vi "main.vi"() -> ()   [LabVIEW 2015]
uses:
  BLE Context/BLE context.lvclass
  ctrls/RefsBox.ctl
  ctrls/QData.ctl
  ctrls/States.ctl
  BLE Message/BLE Message.lvclass
  BLE Context/BLE context.lvclass/BLE context.ctl
panel:
  out "In queue:":i32 caption="Numeric"
  out "Accelerometers":cluster{dbl, dbl, dbl}(graph) caption="Body position:"
  out "HRS Plot":u32(graph) caption="Heart Rate: 102"
  out "Device name":string caption="String"
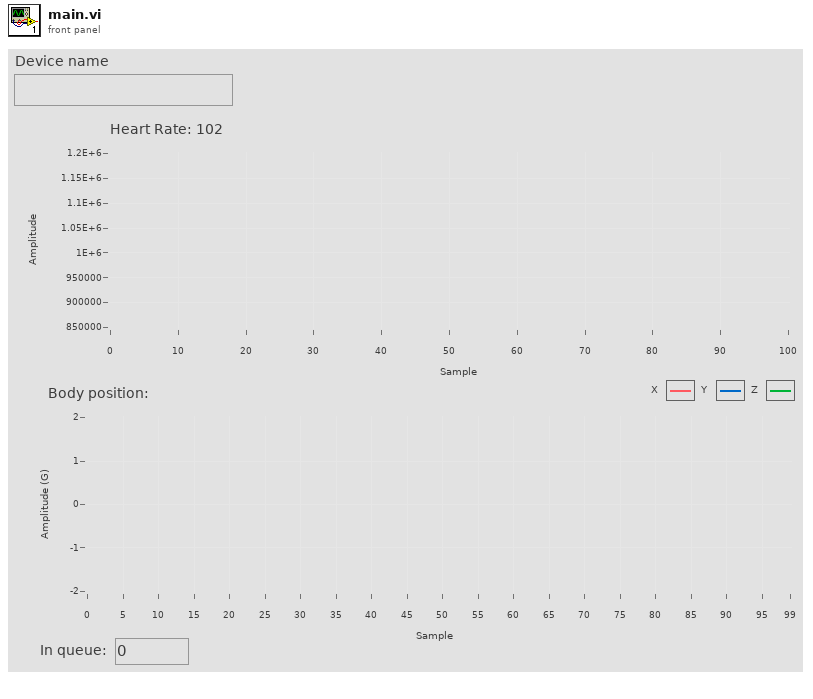
[diagram p1: front panel]
types:
  T1 = typedef "QData.ctl" = cluster{"States":T2, "BLE Message.lvclass":refnum<class "BLE Message.lvclass">}
  T2 = typedef "States.ctl" = enum16{"Stop", "Send"}
  T3 = typedef "RefsBox.ctl" = cluster{"Heart Rate Plot ref":refnum<vi>, "Accelerometers":refnum<vi>, "Main VI":refnum<vi>}
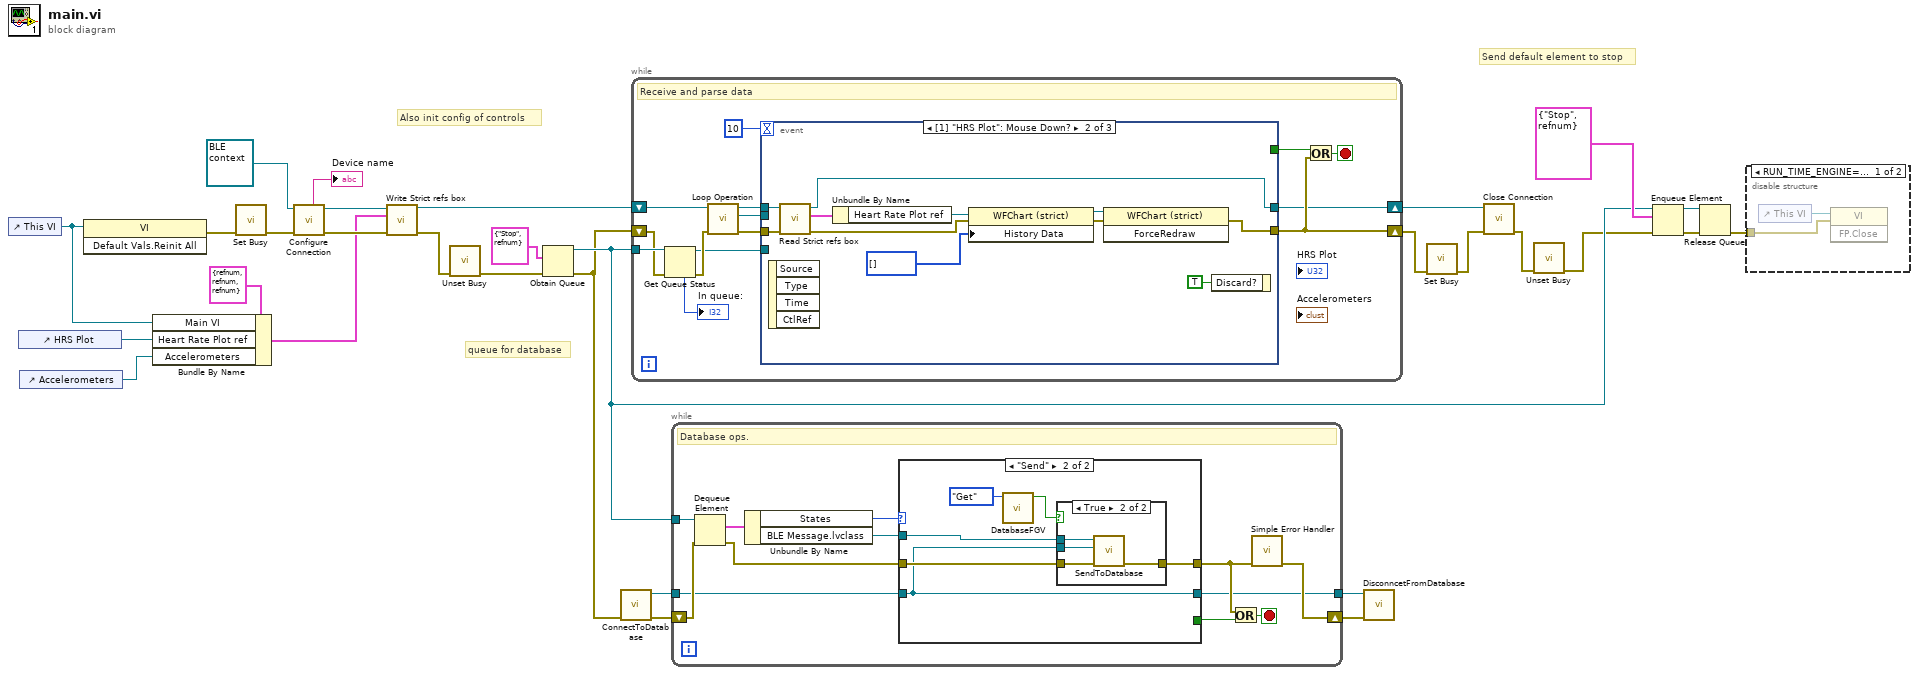
[diagram p0: block diagram]
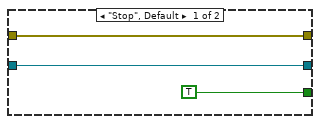
[diagram p3: hidden frame]
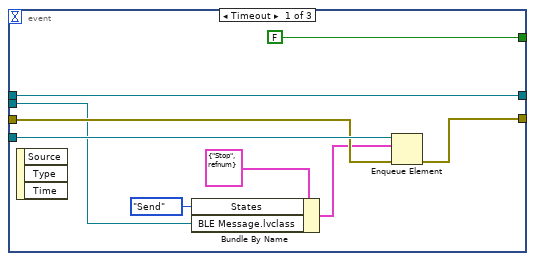
[diagram p5: hidden frame]
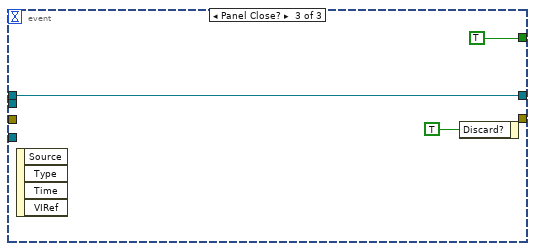
[diagram p6: hidden frame]
diagram:
  # "Send default element to stop"
  # "Also init config of controls"
  # "queue for database"
  n1 = control-ref of="This VI"() -> (w1:refnum<vi>)
  n2 = control-ref of="HRS Plot"() -> (w27:refnum<vi>)
  n3 = control-ref of="Accelerometers"() -> (w21:refnum<vi>)
  n4 = invoke class="VI" method="Default Vals.Reinit All"(reference=w1) -> (error out=w5:errorcluster)  [unwired: 2 in, 2 out]
  n5 = Bundle By Name(cluster=T3 {"Heart Rate Plot ref"=refnum, "Accelerometers"=refnum, "Main VI"=refnum} ("Strict refs box"), "Main VI"=w1, "Heart Rate Plot ref"=w27, "Accelerometers"=w21) -> (w23:T3)
  n6 = call <vilib>:"Set Busy.vi"("error in (no error)"=w5) -> ("error out"=w4:errorcluster)  [unwired: 9 in, 1 out]
  n7 = call "Configure Connection.vi"("error in (no error)"=w4, "BLE context in"=refnum<class "BLE context.lvclass"> refnum ("BLE context.lvclass")) -> ("error out"=w25:errorcluster, "BLE context out"=w26:refnum<class "BLE context.lvclass">, "Device name"=→"Device name":string)  [unwired: 7 in]
  n8 = call "Write Strict refs box.vi"("error in (no error)"=w25, "Strict refs box"=w23, "BLE context in"=w26) -> ("error out"=w3:errorcluster, "BLE context out"=w24:refnum<class "BLE context.lvclass">)  [unwired: 7 in]
  n9 = call <vilib>:"Unset Busy.vi"("error in (no error)"=w3) -> ("error out"=w2:errorcluster)  [unwired: 10 in]
  n10 = Obtain Queue(element data type=T1 {"States"=enum."Stop", "BLE Message.lvclass"=refnum} ("Cluster"), error in (no error)=w2) -> (queue out=w16:refnum<queue>, error out=w14:errorcluster)  [unwired: 3 in, 1 out]
  n11 = call "ConnectToDatabase.vi"("error in"=w14) -> ("error out"=w15:errorcluster, "Database ref"=w13:refnum<k24>)  [unwired: 9 in]
  n12 = while {
    shift-right: [w39] -> w22
    shift-left: w24 -> [w43]
    shift-right: [w40] -> w12
    shift-left: w14 -> [w34]
    tunnel: w16 -> [w35]
    stop <- w44 stop-if-true
    # "Receive and parse data"
    n13 = Get Queue Status(queue=w35, error in (no error)=w34) -> (queue out=w32:refnum<queue>, error out=w33:errorcluster, # elements in queue=→"In queue:":i32)  [unwired: 1 in, 5 out]
    n14 = call "Loop Operation.vi"("error in (no error)"=w33, "BLE context in"=w43) -> ("error out"=w41:errorcluster, "BLE Message out"=w42:refnum<class "BLE Message.lvclass">, "BLE context out"=w38:refnum<class "BLE context.lvclass">)  [unwired: 7 in]
    n15 = event shown="[1] \"HRS Plot\": Mouse Down?" {
      selector: _ -> [_ _ _]
      dyn-events: _ -> [_ _ _]
      timeout: 10 -> [_ _ _]
      tunnel: w42 -> [w47 _ _]
      tunnel: w32 -> [w53 _ _]
      tunnel: w41 -> [w52 w63 _]
      tunnel: [w51 w56 _] -> w40
      tunnel: [w50 w55 w65] -> w39
      tunnel: w38 -> [w50 w64 w65]
      tunnel: [FALSE _ TRUE ("stop? (T)")] -> w36
      event Timeout {
        n16 = event-data() -> ()  [unwired: 1 in, 3 out]
        n17 = Bundle By Name(cluster=T1 {"States"=enum."Stop", "BLE Message.lvclass"=refnum} ("Cluster"), "States"=States."Send", "BLE Message.lvclass"=w47) -> (w45:T1)
        n18 = Enqueue Element(queue=w53, element=w45, error in (no error)=w52) -> (error out=w51:errorcluster)  [unwired: 1 in, 2 out]
      }
      event "HRS Plot": Mouse Down? {
        n19 = event-data() -> ()  [unwired: 1 in, 4 out]
        n20 = call "Read Strict refs box.vi"("error in (no error)"=w63, "BLE context in"=w64) -> ("error out"=w60:errorcluster, "Strict refs box"=w62:T3, "BLE context out"=w55:refnum<class "BLE context.lvclass">)  [unwired: 7 in]
        n21 = Unbundle By Name(w62) -> ("Heart Rate Plot ref"=w61:refnum<vi>)
        n22 = property class="WFChart (strict)"(reference=w61, error in=w60, "History Data"=u32[] []) -> (reference out=w58:refnum<vi>, error out=w57:errorcluster)
        n23 = invoke class="WFChart (strict)" method="ForceRedraw"(reference=w58, error in=w57) -> (error out=w56:errorcluster)  [unwired: 1 in, 2 out]
        n24 = event-data("Discard?"=TRUE) -> ()  [unwired: 1 in, 1 out]
      }
      event Panel Close? {
        n25 = event-data() -> ()  [unwired: 1 in, 4 out]
        n26 = event-data("Discard?"=TRUE) -> ()  [unwired: 1 in, 1 out]
      }
    }
    n27 = Or(x=w36, y=w40) -> (x .or. y?=w44:bool)
  }
  n28 = while {
    tunnel: w16 -> [w79]
    shift-right: [w73] -> w7
    shift-left: w15 -> [w78]
    tunnel: w13 -> [w69]
    tunnel: [w68] -> w8
    stop <- w72 stop-if-true
    # "Database ops."
    n29 = Dequeue Element(queue=w79, error in (no error)=w78) -> (element=w77:T1, error out=w74:errorcluster)  [unwired: 1 in, 2 out]
    n30 = Unbundle By Name(w77) -> ("States"=w76:T2, "BLE Message.lvclass"=w75:refnum<class "BLE Message.lvclass">)
    n31 = case shown="\"Send\"" w76 {
      tunnel: w75 -> [_ w86]
      tunnel: w74 -> [w81 w88]
      tunnel: [TRUE _] -> w71
      tunnel: [w81 w87] -> w70
      tunnel: w69 -> [w80 w85]
      tunnel: [w80 w85] -> w68
      frame "Stop", Default {
      }
      frame "Send" {
        n32 = call "DatabaseFGV.vi"("State"=enum16{"Get", "Set"}."Get") -> ("Active?"=w83:bool)  [unwired: 10 in]
        n33 = case shown="True" w83 {
          tunnel: w88 -> [w89 w93]
          tunnel: [w89 w92] -> w87
          tunnel: w86 -> [_ w91]
          tunnel: w85 -> [_ w90]
          frame False {
          }
          frame True {
            n34 = call "SendToDatabase.vi"("error in (no error)"=w93, "Database ref"=w90, "BLE Message in"=w91) -> ("error out"=w92:errorcluster)  [unwired: 8 in]
          }
        }
      }
    }
    n35 = Or(x=w70, y=w71) -> (x .or. y?=w72:bool)
    n36 = call <vilib>:"Simple Error Handler.vi"("error in (no error)"=w70) -> ("error out"=w73:errorcluster)  [unwired: 4 in, 4 out]
  }
  n37 = call "DisconncetFromDatabase.vi"("error in"=w7, "Database ref"=w8) -> ()  [unwired: 9 in, 1 out]
  n38 = call <vilib>:"Set Busy.vi"("error in (no error)"=w12) -> ("error out"=w11:errorcluster)  [unwired: 9 in, 1 out]
  n39 = call "Close Connection.vi"("error in (no error)"=w11, "BLE context in"=w22) -> ("error out"=w10:errorcluster)  [unwired: 8 in, 1 out]
  n40 = call <vilib>:"Unset Busy.vi"("error in (no error)"=w10) -> ("error out"=w9:errorcluster)  [unwired: 10 in]
  n41 = Enqueue Element(queue=w16, element=T1 {"States"=enum."Stop", "BLE Message.lvclass"=refnum} ("Cluster"), error in (no error)=w9) -> (queue out=w17:refnum<queue>, error out=w18:errorcluster)  [unwired: 1 in, 1 out]
  n42 = Release Queue(queue=w17, error in (no error)=w18) -> (error out=w6:errorcluster)  [unwired: 1 in, 2 out]
  n43 = disable-structure shown="RUN_TIME_ENGINE==True" {
    disable-tunnel: w6 -> [w94 _]
    frame condition #0 {
      n44 = control-ref of="This VI"() -> (w95:refnum<vi>)
      n45 = invoke class="VI" method="FP.Close"(reference=w95, error in=w94) -> ()  [unwired: 1 in, 3 out]
    }
    frame condition #1 (active) {
    }
  }
